vi "WriteLIDARPointToPC.vi"(7 "SelectLIDAR":enum16{"Raphael", "Leonardo"}(ring), 8 "count":u8, 9 "z":i16, 10 "y":i16, 11 "x":i16) -> (2 "Timed Out?":bool)   [LabVIEW 2010]
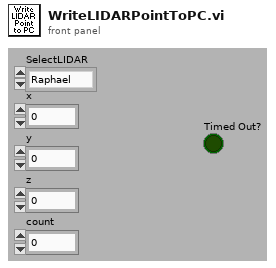
[diagram p1: front panel]
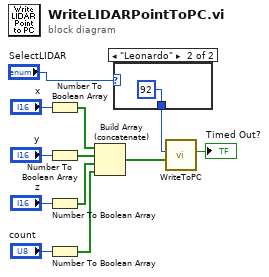
[diagram p0: block diagram]
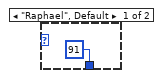
[diagram p2: hidden frame]
diagram:
  n1 = Number To Boolean Array(number="x") -> (Boolean array=w8:bool[])
  n2 = Number To Boolean Array(number="y") -> (Boolean array=w7:bool[])
  n3 = Number To Boolean Array(number="z") -> (Boolean array=w6:bool[])
  n4 = Number To Boolean Array(number="count") -> (Boolean array=w5:bool[])
  n5 = Build Array (concatenate)(w8, w7, w6, w5) -> (w4:bool[])
  n6 = case shown="\"Leonardo\"" "SelectLIDAR" {
    tunnel: [u8 91 ("ID") u8 92 ("ID")] -> w1
    frame "Raphael", Default {
    }
    frame "Leonardo" {
    }
  }
  n7 = call "WriteToPC.vi"("array"=w4, "ID"=w1) -> ("Timed Out?"=→"Timed Out?":bool)  [unwired: 9 in]
